vi "Get Sample Rate.vi"(8 "error in (no error)":errorcluster, 11 "device handle in":T1) -> (0 "error out":errorcluster, 2 "Sample Rate (Hz)":u32, 3 "device handle out":T1)   [LabVIEW 2019, in "RTL-SDR.lvlib"]
uses:
  RTL-SDR.lvlib
  Controls/Device Handle.ctl
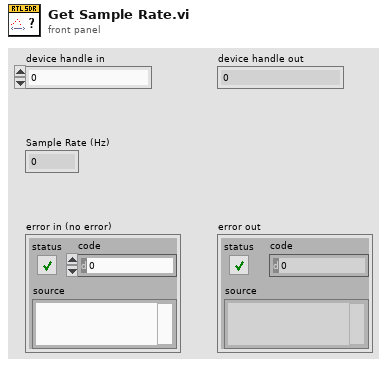
[diagram p1: front panel]
types:
  T1 = typedef "RTL-SDR.lvlib/Device Handle.ctl" = u64
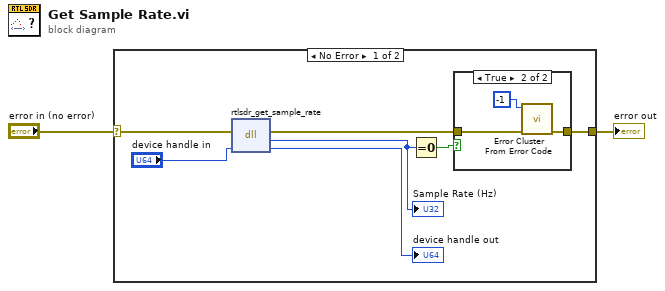
[diagram p0: block diagram]
diagram:
  n1 = case shown="No Error" "error in (no error)" {
    selector: "error in (no error)" -> [w7 w14]
    tunnel: [w5 w14] -> w2
    frame No Error {
      n2 = dll-call lib="usr/local/Cellar/librtlsdr/0.6.0/bin/rtl_sdr" fn="rtlsdr_get_sample_rate"(error in=w7, "dev"="device handle in") -> (error out=w6:errorcluster, "rate"=w4:u32, "dev"=→"device handle out":u64)  [unwired: 2 in, 1 out]
      "Sample Rate (Hz)" <- w4
      n3 = Equal To 0?(x=w4) -> (x = 0?=w3:bool)
      n4 = case shown="True" w3 {
        tunnel: w6 -> [w10 w13]
        tunnel: [w10 w12] -> w5
        frame False {
        }
        frame True {
          n5 = call <vilib>:"Error Cluster From Error Code.vi"("error in (no error)"=w13, "error code (0)"=-1) -> ("error out"=w12:errorcluster)  [unwired: 7 in]
        }
      }
    }
    frame Error {
    }
  }
  "error out" <- w2
